vi "MGCC_MdlMgmt_main_opal_rt.vi"() -> ()   [LabVIEW 2016]
doc: "This VI is the main VI for the model management function. The main purpose of this VI is to initize the input for the state estimation and PQ balancing. Since it will only be run one time, there is no need for the enable button."
uses:
  Finite State Machine/Sub-VIs/MGCC_FntStaMach_gobal.vi
  Communication/MGCC_Global_communication_inputsettings .vi
  <vilib>/Utility/error.llb/Error Cluster From Error Code.vi
  Communication/Global communication output.vi
  Data logging/Sub-Vis/Global tdms reference.vi
  Data logging/Sub-Vis/MGCC_DataLog_global.vi
  Communication/Global communication.vi
  Global_MdlMgmt.vi
  Resynchronization/MGCC_Resync_global.vi
  Abnormal Fault State Control/Sub_VIs/Fault_Abnormal_state.vi
  Planned Islanding/MGCC_PlannedISD_global.vi
  <vilib>/ErrorRing/Error Ring.xnode
  <vilib>/imath/engines/lvmath2/RunTimeEngine/ErrorHandling/NIMS_Finalize Error.vi
  <vilib>/imath/engines/lvmath2/RunTimeEngine/BuiltInFunctions/double/NIMS_double.vi
  <vilib>/imath/engines/lvmath2/RunTimeEngine/NodeEndStatement/NIMS_NodeEndStatement_Output.vi
panel:
  out "x 3":dbl[][](array[numeric])
  out "x 2":dbl[][](array[numeric])
  out "x":dbl[][](array[numeric])
  out "appended array":dbl[](array[numeric])
  out "error out 4":errorcluster
  out "error out 3":errorcluster
  out "error out 2":errorcluster
  out "PV_hist":dbl[](array[numeric])
  # "Copyright <2020> <The University of Tennessee at Knoxville and the University of Tennessee Research Foundation>\n\nRedistribution and use in source and binary forms, with or without modification, are permitted provided that the following conditions are met:\n\n1. Redistributions of source code must retain the above copyright notice, this list of conditions and the following disclaimer.\n\n2. Redistributions in binary form must reproduce the above copyright notice, this list of conditions and the following disclaimer in the documentation and/or other materials provided with the distribution.\n\n3. Neither the name of the copyright holder nor the names of its contributors may be used to endorse or promote products derived from this software without specific prior written permission.\n\nTHIS SOFTWARE IS PROVIDED BY THE COPYRIGHT HOLDERS AND CONTRIBUTORS \"AS IS\" AND ANY EXPRESS OR IMPLIED WARRANTIES, INCLUDING, BUT NOT LIMITED TO, THE IMPLIED WARRANTIES OF MERCHANTABILITY AND FITNESS FOR A PARTICULAR PURPOSE ARE DISCLAIMED. IN NO EVENT SHALL THE COPYRIGHT HOLDER OR CONTRIBUTORS BE LIABLE FOR ANY DIRECT, INDIRECT, INCIDENTAL, SPECIAL, EXEMPLARY, OR CONSEQUENTIAL DAMAGES (INCLUDING, BUT NOT LIMITED TO, PROCUREMENT OF SUBSTITUTE GOODS OR SERVICES; LOSS OF USE, DATA, OR PROFITS; OR BUSINESS INTERRUPTION) HOWEVER CAUSED AND ON ANY THEORY OF LIABILITY, WHETHER IN CONTRACT, STRICT LIABILITY, OR TORT (INCLUDING NEGLIGENCE OR OTHERWISE) ARISING IN ANY WAY OUT OF THE USE OF THIS SOFTWARE, EVEN IF ADVISED OF THE POSSIBILITY OF SUCH DAMAGE."
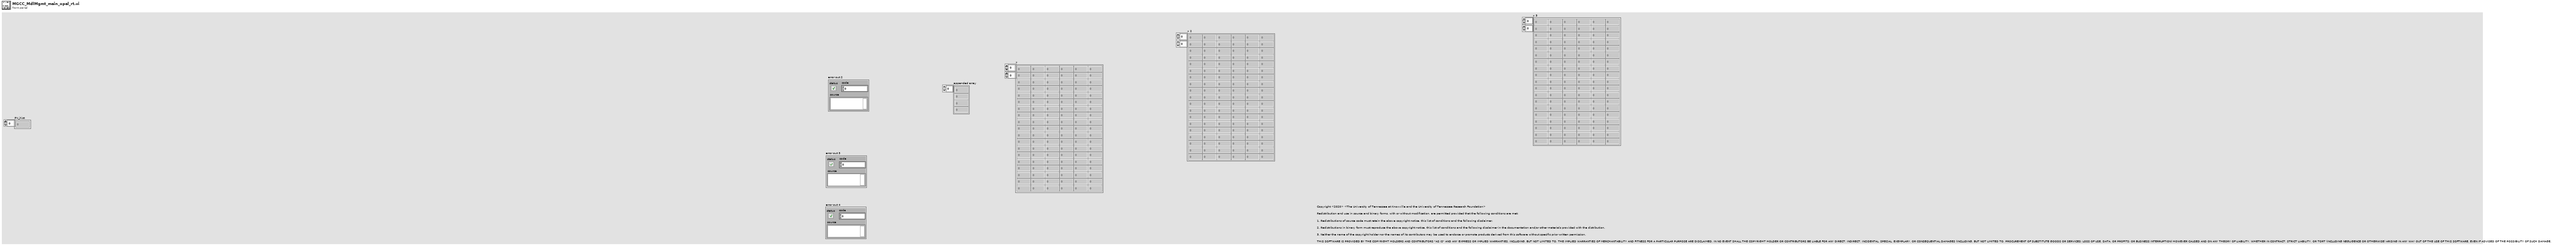
[diagram p1: front panel]
types:
  T1 = enum16{"open", "open or create", "create or replace", "create", "open (read-only)"}
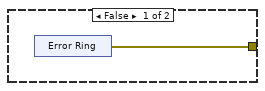
[diagram p2: hidden frame]
diagram:
  n1 = flat-sequence {
    tunnel: [w77] -> w55
    tunnel: [w80] -> w56
    tunnel: w55 -> [w80]
    tunnel: [w79] -> w11
    tunnel: [w82] -> w57
    tunnel: w56 -> [w82]
    tunnel: [w81] -> w12
    tunnel: w11 -> [w81]
    tunnel: [w91] -> w58
    tunnel: w57 -> [w91]
    tunnel: [w87] -> w39
    tunnel: [w86] -> w13
    tunnel: w12 -> [w86]
    tunnel: [w178] -> w59
    tunnel: w58 -> [w178]
    tunnel: [w177] -> w40
    tunnel: w39 -> [w177]
    tunnel: [w176] -> w14
    tunnel: w13 -> [w176]
    tunnel: [w184] -> w60
    tunnel: w59 -> [w184]
    tunnel: [w183] -> w41
    tunnel: w40 -> [w183]
    tunnel: [w182] -> w15
    tunnel: w14 -> [w182]
    tunnel: [w188] -> w61
    tunnel: w60 -> [w188]
    tunnel: [w187] -> w42
    tunnel: w41 -> [w187]
    tunnel: [w186] -> w16
    tunnel: w15 -> [w186]
    tunnel: [w207] -> w62
    tunnel: w61 -> [w207]
    tunnel: [w206] -> w43
    tunnel: w42 -> [w206]
    tunnel: [w205] -> w17
    tunnel: w16 -> [w205]
    tunnel: [w223] -> w63
    tunnel: w62 -> [w223]
    tunnel: [w222] -> w44
    tunnel: w43 -> [w222]
    tunnel: [w221] -> w18
    tunnel: w17 -> [w221]
    tunnel: [w241] -> w64
    tunnel: w63 -> [w241]
    tunnel: [w240] -> w45
    tunnel: w44 -> [w240]
    tunnel: [w239] -> w29
    tunnel: [w238] -> w19
    tunnel: w18 -> [w238]
    tunnel: [w237] -> w1
    tunnel: [w246] -> w65
    tunnel: w64 -> [w246]
    tunnel: [w245] -> w46
    tunnel: w45 -> [w245]
    tunnel: [w244] -> w30
    tunnel: w29 -> [w244]
    tunnel: [w243] -> w20
    tunnel: w19 -> [w243]
    tunnel: [w242] -> w2
    tunnel: w1 -> [w242]
    tunnel: [w251] -> w66
    tunnel: w65 -> [w251]
    tunnel: [w250] -> w47
    tunnel: w46 -> [w250]
    tunnel: [w249] -> w31
    tunnel: w30 -> [w249]
    tunnel: [w248] -> w21
    tunnel: w20 -> [w248]
    tunnel: [w247] -> w3
    tunnel: w2 -> [w247]
    tunnel: [w283] -> w67
    tunnel: w66 -> [w283]
    tunnel: [w282] -> w48
    tunnel: w47 -> [w282]
    tunnel: [w281] -> w32
    tunnel: w31 -> [w281]
    tunnel: [w280] -> w22
    tunnel: w21 -> [w280]
    tunnel: [w279] -> w4
    tunnel: w3 -> [w279]
    tunnel: [w301] -> w68
    tunnel: w67 -> [w301]
    tunnel: [w300] -> w49
    tunnel: w48 -> [w300]
    tunnel: [w299] -> w33
    tunnel: w32 -> [w299]
    tunnel: [w298] -> w23
    tunnel: w22 -> [w298]
    tunnel: [w297] -> w5
    tunnel: w4 -> [w297]
    tunnel: [w308] -> w69
    tunnel: w68 -> [w308]
    tunnel: [w307] -> w50
    tunnel: w49 -> [w307]
    tunnel: [w306] -> w34
    tunnel: w33 -> [w306]
    tunnel: [w305] -> w24
    tunnel: w23 -> [w305]
    tunnel: [w304] -> w6
    tunnel: w5 -> [w304]
    tunnel: [w314] -> w70
    tunnel: w69 -> [w314]
    tunnel: [w313] -> w51
    tunnel: w50 -> [w313]
    tunnel: [w312] -> w35
    tunnel: w34 -> [w312]
    tunnel: [w311] -> w25
    tunnel: w24 -> [w311]
    tunnel: [w310] -> w7
    tunnel: w6 -> [w310]
    tunnel: [w318] -> w71
    tunnel: w70 -> [w318]
    tunnel: [w322] -> w52
    tunnel: w51 -> [w322]
    tunnel: [w321] -> w36
    tunnel: w35 -> [w321]
    tunnel: [w320] -> w26
    tunnel: w25 -> [w320]
    tunnel: [w319] -> w8
    tunnel: w7 -> [w319]
    tunnel: [w328] -> w72
    tunnel: w71 -> [w328]
    tunnel: [w327] -> w53
    tunnel: w52 -> [w327]
    tunnel: [w326] -> w37
    tunnel: w36 -> [w326]
    tunnel: [w325] -> w27
    tunnel: w26 -> [w325]
    tunnel: [w324] -> w9
    tunnel: w8 -> [w324]
    tunnel: [w335] -> w73
    tunnel: w72 -> [w335]
    tunnel: [w334] -> w54
    tunnel: w53 -> [w334]
    tunnel: [w333] -> w38
    tunnel: w37 -> [w333]
    tunnel: [w332] -> w28
    tunnel: w27 -> [w332]
    tunnel: [w331] -> w10
    tunnel: w9 -> [w331]
    tunnel: w73 -> [w340]
    tunnel: w54 -> [w339]
    tunnel: w38 -> [w338]
    tunnel: w28 -> [w337]
    tunnel: w10 -> [w336]
    frame #0 {
      # "The Model Management finish flag initialization"
      n2 = global write "MGCC_FntStaMach_gobal.vi" "b_MGCC_fntStaMach_communication_working"(FALSE ("b_MGCC_fntStaMach_ModelMgmt_done")) -> ()
      n3 = global write "MGCC_FntStaMach_gobal.vi" "b_MGCC_fntStaMach_all_loop_stop"(FALSE ("b_MGCC_fntStaMach_all_loop_stop")) -> ()
      n4 = global write "MGCC_FntStaMach_gobal.vi" "b_MGCC_fntStaMach_ModelMgmt_done"(FALSE ("b_MGCC_fntStaMach_ModelMgmt_done")) -> ()
    }
    frame #1 {
      # "State estimation parts"
      n5 = call "MGCC_StaEst_initial_input_RTDS.vi"() -> ("error out"=w77:errorcluster)  [unwired: 11 in]
      n6 = global write "MGCC_FntStaMach_gobal.vi" "f_MGCC_OnliTopolden_node"(dbl[][] [[1.0, 8.0, 17.0], [2.0, 5.0, 8.0], [3.0, 0.0, 10.0], [0.0, 0.0, 11.0], [0.0, 0.0, 7.0]] ("f_MGCC_OnliTopolden_node")) -> ()
    }
    frame #2 {
      # "FSM flagesm events, states, functions parts"
      n7 = call "MGCC_FntStaMach_Initialization.vi"() -> ("error out"=w79:errorcluster)  [unwired: 11 in]
    }
    frame #3 {
      w83 = FALSE ("S0102-status-ctrl")
      # "switches, irradiance parts"
      n8 = shared-variable "MGCC\\MGCC_FntStaMach_Communication_controls.lvlib\\i_MGCC_FntStaMach_irradiance"(0.0 ("i_MGCC_FntStaMach_irradiance")) -> ()  [unwired: 1 in, 1 out]
      n9 = shared-variable "MGCC\\MGCC_FntStaMach_Finte State Machine.lvlib\\b_MGCC_FntStaMach_readytorun"(FALSE ("b_MGCC_FntStaMach_readytorun")) -> ()  [unwired: 1 in, 1 out]
      n10 = shared-variable "MGCC\\MGCC_BlkStart_Output.lvlib\\b_MGCC_BlkStart_Output_success_flag"(w83) -> ()  [unwired: 1 in, 1 out]
      n11 = shared-variable "MGCC\\MGCC_BlkStart_Output.lvlib\\b_MGCC_BlkStart_Output_failure_flag5"(w83) -> ()  [unwired: 1 in, 1 out]
    }
    frame #4 {
      # "DNP3 Communication"
      n12 = flat-sequence {
        tunnel: [w100] -> w90
        tunnel: [w138] -> w89
        frame #0 {
          n13 = call "MGCC_StaEst_load_complex.vi"("file path (dialog if empty)"=path "c:/model-management/Communication_intellirupters_MGCC.csv" ("file path (use dialog)")) -> ("Array 13"=w101:cdb[][])
          n14 = Empty Array?(array=w101) -> (empty?=w100:bool)
          n15 = Complex To Re/Im(x + iy=w101) -> (x=w124:dbl[][])  [unwired: 1 out]
          "x" <- w124
          n16 = Index Array(array=w124, index (row) #1=1 ("index (row)"), index (col) #1=1 ("disabled index (col)"), index (row) #2=2 ("index (row)"), index (col) #2=1 ("disabled index (col)"), index (row) #3=3 ("index (row)"), index (col) #3=1 ("disabled index (col)"), index (row) #4=4 ("index (row)"), index (col) #4=1 ("disabled index (col)"), index (row) #5=5 ("index (row)"), index (col) #5=1 ("disabled index (col)"), index (row) #6=6 ("index (row)"), index (col) #6=1 ("disabled index (col)"), index (row) #7=7 ("index (row)"), index (col) #7=1 ("disabled index (col)"), index (row) #8=8 ("index (row)"), index (col) #8=1 ("disabled index (col)"), index (row) #9=9 ("index (row)"), index (col) #9=1 ("disabled index (col)"), index (row) #10=10 ("index (row)"), index (col) #10=1 ("disabled index (col)"), index (row) #11=11 ("index (row)"), index (col) #11=1 ("disabled index (col)")) -> (element #1=w134:dbl, element #2=w127:dbl, element #3=w126:dbl, element #4=w125:dbl, element #5=w108:dbl, element #6=w107:dbl, element #7=w106:dbl, element #8=w105:dbl, element #9=w104:dbl, element #10=w103:dbl, element #11=w102:dbl)
          n17 = Build Array(w134, w127, w126, w125) -> (w109:dbl[])
          "appended array" <- w109
          n18 = global write "MGCC_Global_communication_inputsettings .vi" "DNP3 port BESS"(w108) -> ()
          n19 = global write "MGCC_Global_communication_inputsettings .vi" "DNP3 Master Address BESS"(w107) -> ()
          n20 = global write "MGCC_Global_communication_inputsettings .vi" "DNP3 Outstation Address BESS"(w106) -> ()
          n21 = global write "MGCC_Global_communication_inputsettings .vi" "Analogue statues channel number BESS"(w105) -> ()
          n22 = global write "MGCC_Global_communication_inputsettings .vi" "Analogue control channel number BESS"(w104) -> ()
          n23 = global write "MGCC_Global_communication_inputsettings .vi" "Digital statues channel number BESS"(w103) -> ()
          n24 = global write "MGCC_Global_communication_inputsettings .vi" "Digital control channel number BESS"(w102) -> ()
          n25 = global write "MGCC_Global_communication_inputsettings .vi" "IP_BESS"(w109) -> ()
        }
        frame #1 {
          n26 = call "MGCC_StaEst_load_complex.vi"("file path (dialog if empty)"=path "c:/model-management/Communication_intellirupters_MGCC.csv" ("file path (use dialog)")) -> ("Array 13"=w139:cdb[][])
          n27 = Empty Array?(array=w139) -> (empty?=w138:bool)
          n28 = Complex To Re/Im(x + iy=w139) -> (x=w166:dbl[][])  [unwired: 1 out]
          "x 2" <- w166
          n29 = Index Array(array=w166, index (row) #1=1 ("index (row)"), index (col) #1=2 ("disabled index (col)"), index (row) #2=2 ("index (row)"), index (col) #2=2 ("disabled index (col)"), index (row) #3=3 ("index (row)"), index (col) #3=2 ("disabled index (col)"), index (row) #4=4 ("index (row)"), index (col) #4=2 ("disabled index (col)"), index (row) #5=5 ("index (row)"), index (col) #5=2 ("disabled index (col)"), index (row) #6=6 ("index (row)"), index (col) #6=2 ("disabled index (col)"), index (row) #7=7 ("index (row)"), index (col) #7=2 ("disabled index (col)"), index (row) #8=8 ("index (row)"), index (col) #8=2 ("disabled index (col)"), index (row) #9=9 ("index (row)"), index (col) #9=2 ("disabled index (col)"), index (row) #10=10 ("index (row)"), index (col) #10=2 ("disabled index (col)"), index (row) #11=11 ("index (row)"), index (col) #11=2 ("disabled index (col)")) -> (element #1=w151:dbl, element #2=w150:dbl, element #3=w149:dbl, element #4=w148:dbl, element #5=w146:dbl, element #6=w145:dbl, element #7=w144:dbl, element #8=w143:dbl, element #9=w142:dbl, element #10=w141:dbl, element #11=w140:dbl)
          n30 = global write "MGCC_Global_communication_inputsettings .vi" "Analogue statues channel number PV"(w143) -> ()
          n31 = Build Array(w151, w150, w149, w148) -> (w147:dbl[])
          n32 = global write "MGCC_Global_communication_inputsettings .vi" "Analogue control channel number PV"(w142) -> ()
          n33 = global write "MGCC_Global_communication_inputsettings .vi" "Digital statues channel number PV"(w141) -> ()
          n34 = global write "MGCC_Global_communication_inputsettings .vi" "Digital control channel number PV"(w140) -> ()
          n35 = global write "MGCC_Global_communication_inputsettings .vi" "DNP3 Outstation Address PV"(w144) -> ()
          n36 = global write "MGCC_Global_communication_inputsettings .vi" "DNP3 Master Address PV"(w145) -> ()
          n37 = global write "MGCC_Global_communication_inputsettings .vi" "DNP3 port PV"(w146) -> ()
          n38 = global write "MGCC_Global_communication_inputsettings .vi" "IP_PV"(w147) -> ()
        }
      }
      n39 = Or(x=w90, y=w89) -> (x .or. y?=w88:bool)
      n40 = case shown="True" w88 {
        tunnel: [w92 w94] -> w87
        frame False {
          n41 = xnode "Error Ring"() -> ("error out"=w92:errorcluster)
        }
        frame True {
          n42 = xnode "Error Ring"() -> ("error out"=w94:errorcluster)
        }
      }
    }
    frame #5 {
      n43 = call "MGCC_StaEst_load_complex.vi"("file path (dialog if empty)"=path "c:/model-management/LC_comm.csv" ("file path (use dialog)")) -> ("Array 13"=w180:cdb[][])
      n44 = Complex To Re/Im(x + iy=w180) -> (x=w179:dbl[][])  [unwired: 1 out]
      "x 3" <- w179
      n45 = global write "Global communication output.vi" "comm_matrix"(w179) -> ()
    }
    frame #6 {
      # "BKS & PQ"
      n46 = shared-variable "MGCC\\MGCC_BlkStart_Output.lvlib\\b_MGCC_BlkStart_Output_failure_flag5"(FALSE) -> ()  [unwired: 1 in, 1 out]
    }
    frame #7 {
      # "PV forecasting"
      n47 = disable-structure shown="Disabled" {
        frame Disabled {
          n48 = mathscript code="PV_hist=double(zeros(88,1));"() -> ("PV_hist"=w189:dbl[])  [unwired: 1 in, 1 out]
          "PV_hist" <- w189
          n49 = shared-variable "MGCC\\MGCC_PVFcst_dataIO.lvlib\\f_MGCC_PVFcst_HistoricalPV_sunny"(w189) -> ()  [unwired: 1 in, 1 out]
        }
        frame Enabled {
        }
      }
    }
    frame #8 {
      (unwired) errorcluster {"status"=FALSE, "code"=0, "source"=""} ("e_MGCC_StaEst_error")
      (unwired) errorcluster {"status"=FALSE, "code"=0, "source"=""} ("error in (no error)")
      (unwired) errorcluster {"status"=FALSE, "code"=0, "source"=""} ("e_MGCC_EnergyMgmt_error")
      (unwired) errorcluster {"status"=FALSE, "code"=0, "source"=""} ("error in (no error)")
      (unwired) errorcluster {"status"=FALSE, "code"=0, "source"=""} ("e_MGCC_LoadFcst_error")
      (unwired) cluster{"status":bool} {"status"=FALSE} ("e_MGCC_ProtCoord_error")
      (unwired) errorcluster {"status"=FALSE, "code"=0, "source"=""} ("error in (no error)")
      (unwired) errorcluster {"status"=FALSE, "code"=0, "source"=""} ("e_MGCC_PQBal_error")
      (unwired) errorcluster {"status"=FALSE, "code"=0, "source"=""} ("e_MGCC_Commun_error")
      # "error state control"
      n50 = shared-variable "MGCC\\MGCC_FntStaMach_Finte State Machine.lvlib\\e_MGCC_FntStaMach_Error"(errorcluster {"status"=FALSE, "code"=0, "source"=""} ("e_MGCC_FntStaMach_Error"), error in=errorcluster {"status"=FALSE, "code"=0, "source"=""} ("error in (no error)")) -> ()  [unwired: 1 out]
      n51 = shared-variable "MGCC\\MGCC.lvlib\\e_MGCC_DataLog_error"(errorcluster {"status"=FALSE, "code"=0, "source"=""} ("e_MGCC_DataLog_error"), error in=errorcluster {"status"=FALSE, "code"=0, "source"=""} ("error in (no error)")) -> ()  [unwired: 1 out]
      n52 = shared-variable "MGCC\\MGCC_Resync.lvlib\\e_MGCC_Resync_error"(errorcluster {"status"=FALSE, "code"=0, "source"=""} ("e_MGCC_Resync_error"), error in=errorcluster {"status"=FALSE, "code"=0, "source"=""} ("error in (no error)")) -> ()  [unwired: 1 out]
      n53 = shared-variable "MGCC\\MGCC_MdlMgmt.lvlib\\e_MGCC_MdlMgmt_error"(errorcluster {"status"=FALSE, "code"=0, "source"=""} ("e_MGCC_MdlMgmt_error"), error in=errorcluster {"status"=FALSE, "code"=0, "source"=""} ("error in (no error)")) -> ()  [unwired: 1 out]
      n54 = shared-variable "MGCC\\MGCC_comm_lib.lvlib\\e_MGCC_Commun_error"(errorcluster {"status"=FALSE, "code"=0, "source"=""} ("error in (no error)")) -> ()  [unwired: 1 in, 1 out]
      n55 = shared-variable "MGCC\\MGCC_BlkStart_Output.lvlib\\e_MGCC_BlkStart_error"(errorcluster {"status"=FALSE, "code"=0, "source"=""} ("e_MGCC_BlkStart_error"), error in=errorcluster {"status"=FALSE, "code"=0, "source"=""} ("error in (no error)")) -> ()  [unwired: 1 out]
      n56 = shared-variable "MGCC\\MGCC_StaEst.lvlib\\e_MGCC_StaEst_error"(errorcluster {"status"=FALSE, "code"=0, "source"=""} ("e_MGCC_StaEst_error"), error in=errorcluster {"status"=FALSE, "code"=0, "source"=""} ("error in (no error)")) -> ()  [unwired: 1 out]
    }
    frame #9 {
      # "Data logging"
      n57 = global write "MGCC_DataLog_global.vi" "Sampling step"(100.0 ("Sampling step")) -> ()
      n58 = TDMS Open(10:T1."create or replace" ("operation (0:open)"), 11:path "c:/datalogging/PV_LC_datalog" ("file path (dialog if empty)")) -> (0:→"error out 4":errorcluster, 3:w225:refnum<k34>)  [unwired: 5 in]
      n59 = TDMS Open(10:T1."create or replace" ("operation (0:open)"), 11:path "c:/datalogging/Switch_datalog" ("file path (dialog if empty)")) -> (0:→"error out 3":errorcluster, 3:w229:refnum<k34>)  [unwired: 5 in]
      n60 = global write "Global tdms reference.vi" "Switch tdms file out"(w229) -> ()
      n61 = TDMS Open(10:T1."create or replace" ("operation (0:open)"), 11:path "c:/datalogging/Batt_LC_datalog" ("file path (dialog if empty)")) -> (0:→"error out 2":errorcluster, 3:w233:refnum<k34>)  [unwired: 5 in]
      n62 = global write "Global tdms reference.vi" "Batt tdms file out"(w233) -> ()
      n63 = global write "Global tdms reference.vi" "PV tdms file out"(w225) -> ()
    }
    frame #10 {
      n64 = call "MGCC_MdlMgmt_MovetonewMicrogrid.vi"() -> ("error out"=w239:errorcluster, "error out 2"=w237:errorcluster)  [unwired: 10 in]
    }
    frame #11 {
      n65 = call "MGCC_MdlMgmt_converttopology.vi"() -> ()  [unwired: 12 in]
    }
    frame #12 {
      n66 = Initialize Array(0.0 ("element"), 10 ("dimension size")) -> (w264:dbl[])
      n67 = Initialize Array(0.0 ("element"), 10 ("dimension size")) -> (w258:dbl[])
      n68 = Initialize Array(0.0 ("element"), 10 ("dimension size")) -> (w271:dbl[])
      n69 = Initialize Array(0.0 ("element"), 30 ("dimension size")) -> (w255:dbl[])
      n70 = Initialize Array(0.0 ("element"), 10 ("dimension size")) -> (w266:dbl[])
      n71 = Initialize Array(FALSE, 8 ("dimension size")) -> (w253:bool[])
      n72 = Initialize Array(0.0 ("element"), 10 ("dimension size")) -> (w265:dbl[])
      n73 = Initialize Array(0.0 ("element"), 10 ("dimension size")) -> (w261:dbl[])
      n74 = global write "Global communication output.vi" "LC1 Control"(w255) -> ()
      n75 = global write "Global communication output.vi" "BESS1 Control"(w264) -> ()
      n76 = global write "Global communication output.vi" "LC2 Control"(w258) -> ()
      n77 = global write "Global communication output.vi" "IntellRupter Control"(w253) -> ()
      n78 = global write "Global communication output.vi" "PV Control"(w271) -> ()
      n79 = global write "Global communication.vi" "PV LC communication"(w265) -> ()
      n80 = global write "Global communication.vi" "BESS LC communication"(w266) -> ()
      n81 = global write "Global communication output.vi" "BESS2 Control"(w261) -> ()
    }
    frame #13 {
      n82 = Initialize Array(0.0 ("element"), 10 ("dimension size")) -> (w286:dbl[])
      n83 = global read "Global_MdlMgmt.vi" "Switch number"() -> (w278:dbl)
      n84 = global write "Global communication.vi" "BESS APF ave"(0.0 ("BESS APF ave")) -> ()
      n85 = Add(x=2.0, y=w278) -> (x+y=w277:dbl)
      n86 = global write "Global communication.vi" "BESS APF 1 s"(w286) -> ()
      n87 = global write "Global communication.vi" "PV APF ave"(0.0 ("PV APF ave")) -> ()
      n88 = Initialize Array(0.0 ("element"), w278) -> (w291:dbl[])
      n89 = global write "Global communication.vi" "PV APF 1 s"(w286) -> ()
      n90 = Initialize Array(0.0 ("element"), 10 ("dimension size"), w278) -> (w290:dbl[][])
      n91 = Initialize Array(FALSE, w277) -> (w294:bool[])
      n92 = global write "Global communication.vi" "APF average"(w291) -> ()
      n93 = global write "Global communication.vi" "APF 1s"(w290) -> ()
      n94 = global write "Global communication output.vi" "IntellRupter Control"(w294) -> ()
    }
    frame #14 {
      n95 = disable-structure shown="Disabled" {
        frame Disabled {
          n96 = global read "Global_MdlMgmt.vi" "Switch number"() -> ()  [unwired: 1 out]
        }
        frame Enabled {
        }
      }
      n97 = Initialize Array(0.0 ("element"), 10 ("dimension size")) -> (w302:dbl[])
      n98 = global write "Global communication.vi" "APF"(w302) -> ()
      n99 = global write "Global communication.vi" "FREQ-L"(w302) -> ()
      n100 = global write "Global communication.vi" "FREQ-R"(w302) -> ()
      n101 = global write "Global communication.vi" "MAG-A-L"(w302) -> ()
      n102 = global write "Global communication.vi" "MAG-A-R"(w302) -> ()
      n103 = global write "Global communication.vi" "MAG-B-L"(w302) -> ()
      n104 = global write "Global communication.vi" "MAG-B-R"(w302) -> ()
      n105 = global write "Global communication.vi" "MAG-C-L"(w302) -> ()
      n106 = global write "Global communication.vi" "MAG-C-R"(w302) -> ()
      n107 = global write "Global communication.vi" "RPF"(w302) -> ()
      n108 = global write "Global communication.vi" "Status"(w302) -> ()
      n109 = global write "Global communication.vi" "Reserved13"(w302) -> ()
      n110 = global write "Global communication.vi" "Reserved14"(w302) -> ()
      n111 = global write "Global communication.vi" "Reserved15"(w302) -> ()
      n112 = global write "Global communication.vi" "ANG-DIFF"(w302) -> ()
    }
    frame #15 {
      # "Model management Done flag"
      n113 = shared-variable "MGCC\\MGCC_MdlMgmt.lvlib\\b_MGCC_MdlMgmt_done"(TRUE ("b_MGCC_MdlMgmt_done")) -> ()  [unwired: 1 in, 1 out]
    }
    frame #16 {
      n114 = Initialize Array(FALSE ("b_MGCC_MdlMgmt_done"), 2 ("dimension size")) -> (w317:bool[])
      n115 = global write "MGCC_Resync_global.vi" "b_MGCC_Resync_Enable"(w317) -> ()
    }
    frame #17 {
    }
    frame #18 {
      (unwired) bool[] [TRUE, TRUE, TRUE, TRUE, TRUE, TRUE, TRUE, TRUE, TRUE, TRUE, TRUE] ("Function enable by fault/abnormal")
      w329 = bool[] [FALSE, FALSE]
      # "Fault and abnormal state control"
      n116 = global write "MGCC_FntStaMach_gobal.vi" "Function enable by fault/abnormal"(bool[][] [[TRUE, TRUE, TRUE, TRUE, TRUE, TRUE, TRUE, TRUE, TRUE, TRUE, TRUE], [TRUE, TRUE, FALSE, FALSE, FALSE, FALSE, FALSE, FALSE, FALSE, FALSE, FALSE], [TRUE, TRUE, FALSE, FALSE, FALSE, FALSE, FALSE, FALSE, FALSE, FALSE, FALSE], [TRUE, TRUE, FALSE, FALSE, FALSE, FALSE, FALSE, FALSE, FALSE, FALSE, FALSE], [TRUE, TRUE, FALSE, FALSE, FALSE, FALSE, FALSE, FALSE, FALSE, FALSE, FALSE], [TRUE, TRUE, FALSE, FALSE, FALSE, FALSE, FALSE, FALSE, FALSE, FALSE, FALSE], [TRUE, TRUE, FALSE, FALSE, FALSE, FALSE, FALSE, FALSE, FALSE, FALSE, FALSE], [TRUE, TRUE, FALSE, FALSE, FALSE, FALSE, FALSE, FALSE, FALSE, FALSE, FALSE], [TRUE, TRUE, FALSE, FALSE, FALSE, FALSE, FALSE, FALSE, FALSE, FALSE, FALSE], [TRUE, TRUE, FALSE, FALSE, FALSE, FALSE, FALSE, FALSE, FALSE, FALSE, FALSE], [TRUE, TRUE, FALSE, FALSE, FALSE, FALSE, FALSE, FALSE, FALSE, FALSE, FALSE]] ("Function enable by fault/abnormal")) -> ()
      n117 = global write "Fault_Abnormal_state.vi" "Abnormal state flag"(w329) -> ()
      n118 = global write "Fault_Abnormal_state.vi" "Fault state flag"(w329) -> ()
    }
    frame #19 {
      # "Load calculation"
      n119 = global write "MGCC_PlannedISD_global.vi" "Grid_interface"(1.0 ("Grid")) -> ()
    }
    frame #20 {
      n120 = Merge Errors(w340, w339, w338, w337, w336) -> (w341:errorcluster)
      n121 = global write "Fault_Abnormal_state.vi" "e_MGCC_MdlMgmt_error"(w341) -> ()
    }
    frame #21 {
      n122 = global write "MGCC_FntStaMach_gobal.vi" "b_MGCC_fntStaMach_ModelMgmt_done"(TRUE ("b_MGCC_fntStaMach_ModelMgmt_done")) -> ()
    }
  }
